vi "EndAction.vi"(6 "StartTime":timestamp, 11 "Array":string[](array[string])) -> (0 "Current Time":dbl, 3 "Enqueue":string)   [LabVIEW 2019, in "Scripts.lvclass"]
uses:
  Scripts.lvclass
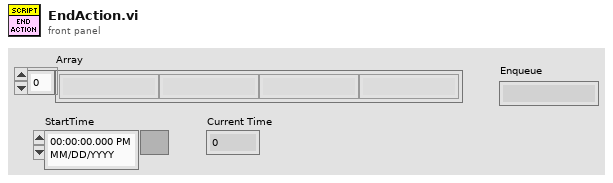
[diagram p1: front panel]
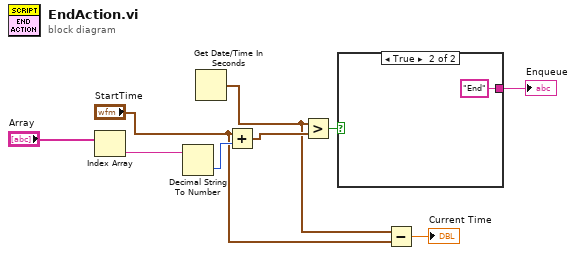
[diagram p0: block diagram]
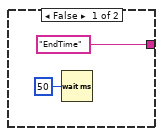
[diagram p2: hidden frame]
diagram:
  n1 = Index Array(array="Array") -> (element=w8:string)  [unwired: 1 in]
  n2 = Decimal String To Number(string=w8) -> (number=w7:i32)  [unwired: 2 in, 1 out]
  n3 = Get Date/Time In Seconds() -> (seconds since 1Jan1904=w1:timestamp)
  n4 = Add(x="StartTime", y=w7) -> (x+y=w4:timestamp)
  n5 = Greater?(x=w1, y=w4) -> (0:w6:bool)
  n6 = case shown="True" w6 {
    tunnel: ["EndTime" ("element") "End" ("element")] -> w5
    frame False {
      n7 = Wait (ms)(milliseconds to wait=u32 50) -> ()  [unwired: 1 out]
    }
    frame True {
    }
  }
  "Enqueue" <- w5
  n8 = Subtract(x=w1, y="StartTime") -> (x-y=→"Current Time":dbl)
